vi "build2Dwaveform(SubVI).vi"(2 "Volt/Div Ch 2":dbl(ring)=1.0 items=["10V"=10.0, "5V"=5.0, "2V"=2.0, "1V"=1.0, "500mV"=0.5, "200mV"=0.2, "100mV"=0.1, "50mV"=0.05, "20mV"=0.02, "10mV"=0.01], 3 "Volt/Div Ch 1":dbl(ring)=1.0 items=["10V"=10.0, "5V"=5.0, "2V"=2.0, "1V"=1.0, "500mV"=0.5, "200mV"=0.2, "100mV"=0.1, "50mV"=0.05, "20mV"=0.02, "10mV"=0.01], 4 "Array":dbl[][](array[numeric]), 5 "waveform":waveform(dbl)) -> (0 "secondo segnale":waveform(dbl)(graph), 1 "primo segnale":waveform(dbl)(graph))   [LabVIEW 2018]
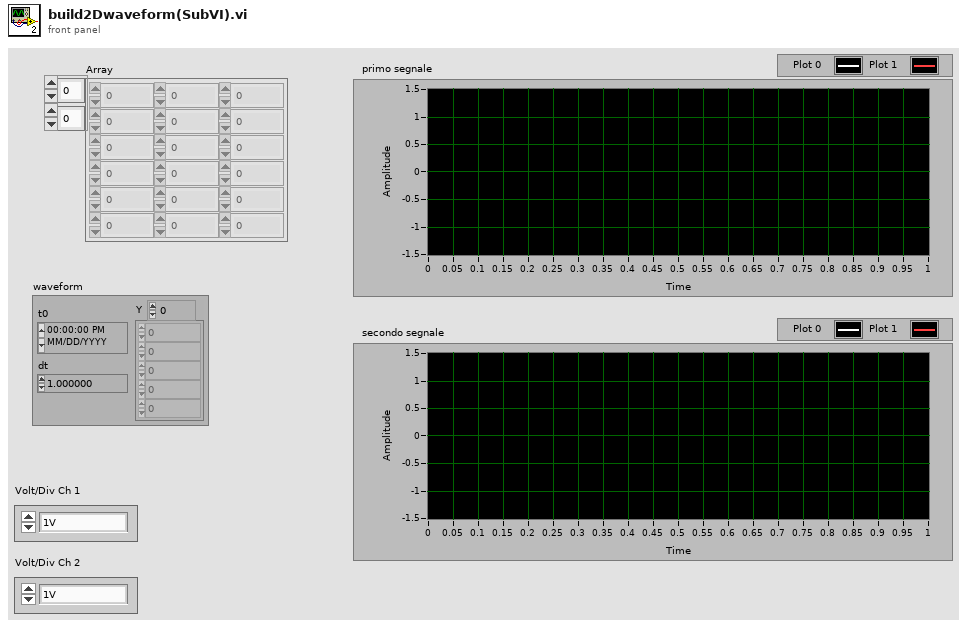
[diagram p1: front panel]
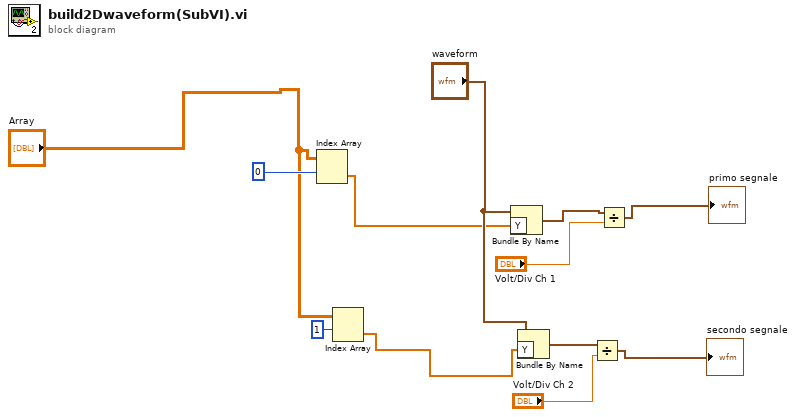
[diagram p0: block diagram]
diagram:
  n1 = Index Array(array="Array", index (row)=0) -> (element=w7:dbl[])  [unwired: 1 in]
  n2 = Index Array(array="Array", index (row)=1) -> (element=w9:dbl[])  [unwired: 1 in]
  n3 = Bundle By Name(cluster="waveform", "Y"=w7) -> (w6:waveform(dbl))
  n4 = Bundle By Name(cluster="waveform", "Y"=w9) -> (w3:waveform(dbl))
  n5 = Divide(x=w3, y="Volt/Div Ch 2") -> (x/y=→"secondo segnale":waveform(dbl))
  n6 = Divide(x=w6, y="Volt/Div Ch 1") -> (x/y=→"primo segnale":waveform(dbl))
